vi "FTW-Scripter-Launch.vi"(5 "My Data":bool, 9 "Timeout":i32=-2 format="%d msec", 11 "error in":errorcluster) -> (4 "FTW Actor Connector":refnum<class "FTW-ActorConnector.lvclass">, 6 "Initialized Response":string, 8 "Instance Inbox Address":string, 15 "error out":errorcluster)   [LabVIEW 2015]
uses:
  source/actor/Connector/FTW-ActorConnector.lvclass
  core/FTW-Scripter-Core_Process.vi
  core/FTW-Scripter-Core.lvclass
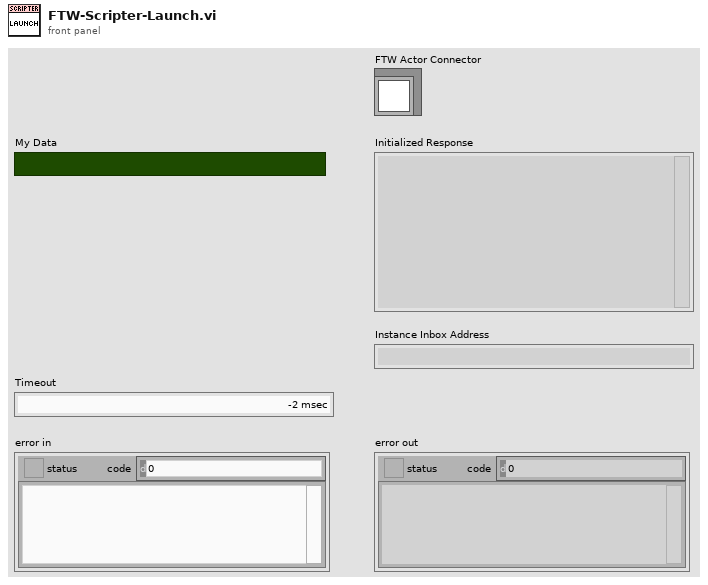
[diagram p1: front panel]
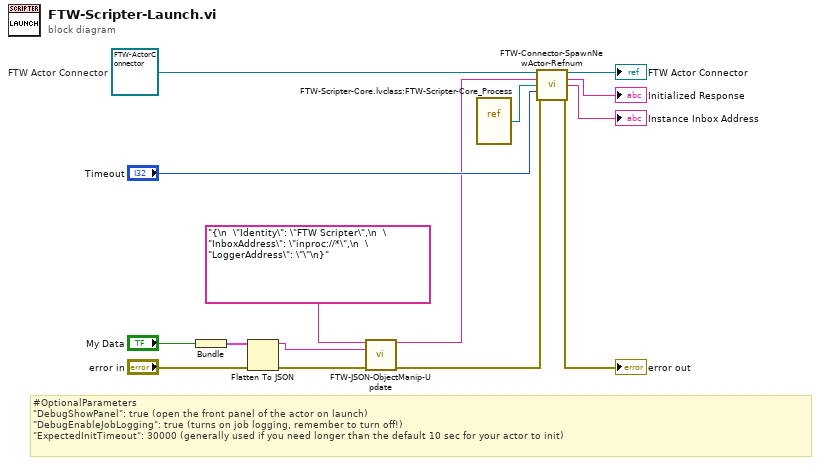
[diagram p0: block diagram]
diagram:
  w15 = refnum<class "FTW-ActorConnector.lvclass"> refnum  # FTW Actor Connector
  # "#OptionalParameters\n\"DebugShowPanel\": true (open the front panel of the actor on launch)\n\"DebugEnableJobLogging\": true (turns on job logging, remember to turn off!)\n\"ExpectedInitTimeout\": 30000 (generally used if you need longer than the default 10 sec for your actor to init)"
  n1 = Bundle("My Data"="My Data") -> (w7:cluster{"My Data":bool})  [unwired: 1 in]
  n2 = Flatten To JSON(anything=w7, error in (no error)="error in") -> (JSON string=w4:string, 11:w6:errorcluster)  [unwired: 1 in]
  n3 = call "FTW-JSON-ObjectManip-Update.vi"("Input JSON Object"="{\n  \"Identity\": \"FTW Scripter\",\n  \"InboxAddress\": \"inproc://*\",\n  \"LoggerAddress\": \"\"\n}" ("Configuration"), "JSON Object to Merge"=w4, "error in"=w6) -> ("Output JSON Object"=w3:string, "error out"=w2:errorcluster)  [unwired: 11 in]
  n4 = vi-ref "FTW-Scripter-Core.lvclass:FTW-Scripter-Core_Process.vi"() -> (w1:refnum<vi>)
  n5 = call "FTW-Connector-SpawnNewActor-Refnum.vi"("FTW Actor Connector Type"=w15, "Configuration"=w3, "Actor VI Refnum"=w1, "Timeout"="Timeout", "error in"=w2) -> ("FTW Actor Connector"=→"FTW Actor Connector":refnum<class "FTW-ActorConnector.lvclass">, "Initialized Response"=→"Initialized Response":string, "Instance Inbox Address"=→"Instance Inbox Address":string, "error out"=→"error out":errorcluster)  [unwired: 7 in]
